vi "Create.vi"(8 "error in (no error)":errorcluster, 9 "Task ID":string, 10 "EnQr":refnum<class "Message Enqueuer.lvclass">) -> (0 "error out":errorcluster, 3 "DataHandlerAPI out":refnum<class "DataHandlerAPI.lvclass">)   [LabVIEW 2020, in "Volatus.lvlib" / "DataHandlerAPI.lvclass"]
uses:
  DataHandlerAPI.lvclass
  <vilib>/ActorFramework/Message Enqueuer/Message Enqueuer.lvclass
  DataHandlerAPI.lvclass/DataHandlerAPI.ctl
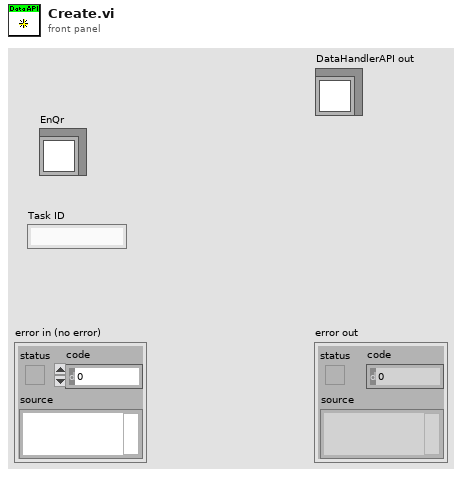
[diagram p1: front panel]
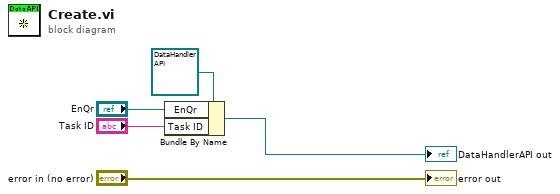
[diagram p0: block diagram]
diagram:
  n1 = Bundle By Name(cluster=refnum<class "DataHandlerAPI.lvclass"> refnum ("DataHandlerAPI in"), "EnQr"="EnQr", "Task ID"="Task ID") -> (→"DataHandlerAPI out":refnum<class "DataHandlerAPI.lvclass">)
  "error out" <- "error in (no error)"
